vi "MSEncoder Case-7-AcqSig.vi"(8 "error in (no error)":errorcluster, 9 "ParamValIn":variant, 11 "MSEncoder in":refnum<class "MSEncoder.lvclass">) -> (0 "error out":errorcluster, 3 "MSEncoder out":refnum<class "MSEncoder.lvclass">)   [LabVIEW 2018, in "MSEncoder.lvclass"]
uses:
  MSEncoder.lvclass
  Ctl/MSEditorParam acqSig.ctl
  MSEncoder.lvclass/MSEncoder.ctl
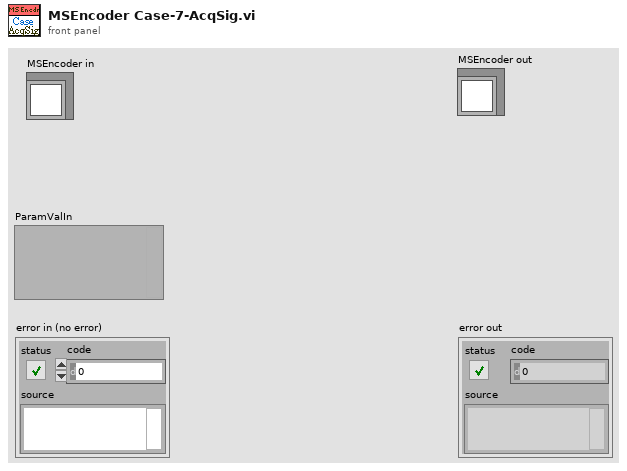
[diagram p1: front panel]
types:
  T1 = typedef "MSEditorParam acqSig.ctl" = cluster{"time ":dbl}
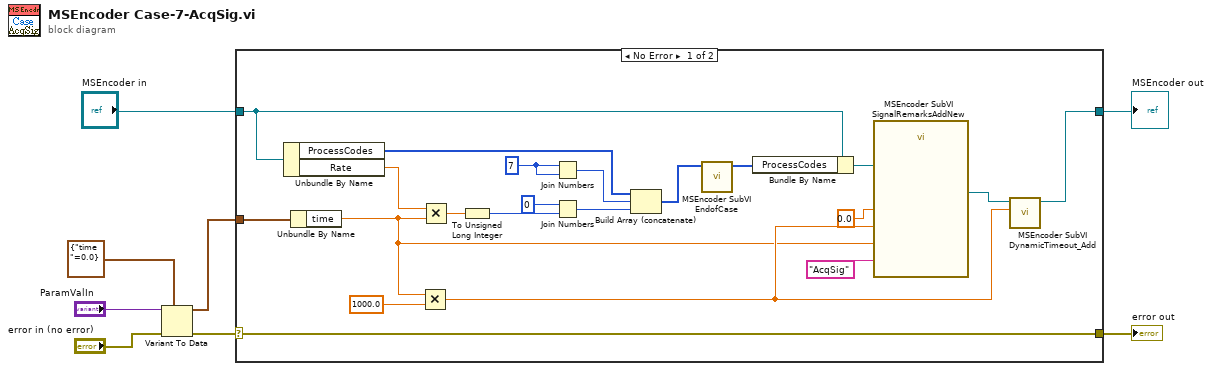
[diagram p0: block diagram]
diagram:
  n1 = Variant To Data(error in="error in (no error)", type=T1 {"time "=0.0} ("ParamValueType"), Variant="ParamValIn") -> (data=w3:T1, error out=w2:errorcluster)
  n2 = case shown="No Error" w2 {
    selector: w2 -> [w28 w31]
    tunnel: "MSEncoder in" -> [w27 w30]
    tunnel: [w28 w31] -> w8
    tunnel: [w22 w30] -> w6
    tunnel: w3 -> [w23 _]
    frame No Error {
      w25 = u32 7
      n3 = Unbundle By Name(w27) -> ("ProcessCodes"=w29:u64[], "Rate"=w21:dbl)
      n4 = Unbundle By Name(w23) -> ("time"=w10:dbl)
      n5 = Multiply(x=w10, y=1000.0) -> (x*y=w11:dbl)
      n6 = Multiply(x=w21, y=w10) -> (x*y=w14:dbl)
      n7 = To Unsigned Long Integer(number=w14) -> (unsigned 32bit integer=w19:u32)
      n8 = Join Numbers(hi=w25, lo=w25) -> ((hi.lo)=w20:u64)
      n9 = Join Numbers(hi=u32 0, lo=w19) -> ((hi.lo)=w17:u64)
      n10 = Build Array (concatenate)(w29, w20, w17) -> (w24:u64[])
      n11 = call "MSEncoder SubVI EndofCase.vi"("Case codes"=w24) -> ("Case codes with end"=w26:u64[])  [unwired: 9 in, 1 out]
      n12 = Bundle By Name(cluster=w27, "ProcessCodes"=w26) -> (w13:refnum<class "MSEncoder.lvclass">)
      n13 = call "MSEncoder SubVI SignalRemarksAddNew.vi"("Label"="AcqSig", "Scan time"=w10, "mz 1"=0.0 ("mz 0"), "mz 0"=w11, "MSEncoder in"=w13) -> ("MSEncoder out"=w15:refnum<class "MSEncoder.lvclass">)  [unwired: 5 in, 1 out]
      n14 = call "MSEncoder SubVI DynamicTimeout_Add.vi"("Timeout_ms"=w11, "MSEncoder"=w15) -> ("MSEncoder"=w22:refnum<class "MSEncoder.lvclass">)  [unwired: 8 in, 1 out]
    }
    frame Error {
    }
  }
  "error out" <- w8
  "MSEncoder out" <- w6
